vi "RT Main.vi"() -> ()   [LabVIEW 2016]
panel:
  out "dequeued element":i32
  out "elements in queue":i32[](array[numeric])
  out "# elements in queue":i32
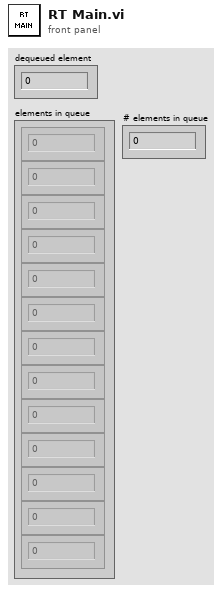
[diagram p1: front panel]
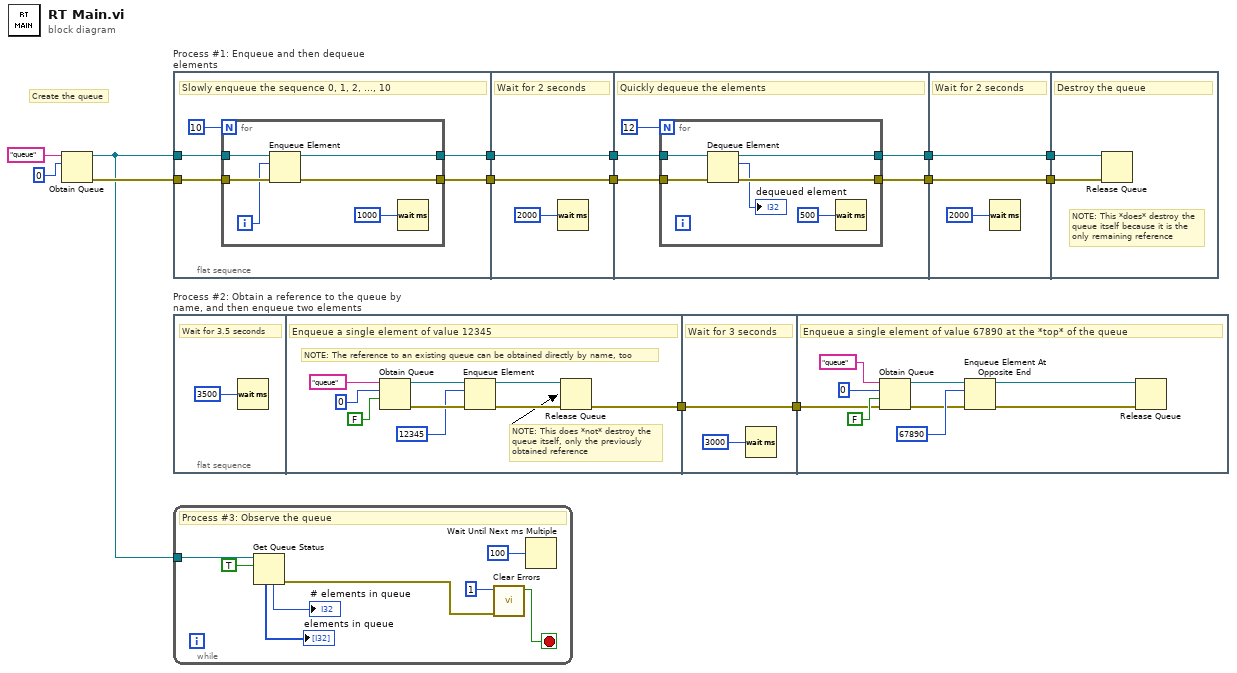
[diagram p0: block diagram]
diagram:
  # "Create the queue"
  n1 = Obtain Queue(name (unnamed)="queue", element data type=0) -> (queue out=w11:refnum<queue>, error out=w12:errorcluster)  [unwired: 3 in, 1 out]
  n2 = flat-sequence "Process #1: Enqueue and then dequeue elements" {
    tunnel: w12 -> [w19]
    tunnel: w11 -> [w17]
    tunnel: [w16] -> w8
    tunnel: [w15] -> w7
    tunnel: w8 -> [w27]
    tunnel: [w27] -> w6
    tunnel: w7 -> [w26]
    tunnel: [w26] -> w5
    tunnel: w6 -> [w29]
    tunnel: w5 -> [w30]
    tunnel: [w32] -> w4
    tunnel: [w31] -> w3
    tunnel: w4 -> [w42]
    tunnel: w3 -> [w41]
    tunnel: [w42] -> w2
    tunnel: [w41] -> w1
    tunnel: w2 -> [w44]
    tunnel: w1 -> [w43]
    frame #0 {
      # "Slowly enqueue the sequence 0, 1, 2, ..., 10"
      n3 = for {
        N: 10 -> [_]
        tunnel: w19 -> [w25]
        tunnel: w17 -> [w24]
        tunnel: [w21] -> w15
        tunnel: [w20] -> w16
        i -> [w23]
        n4 = Enqueue Element(queue=w24, element=w23, error in (no error)=w25) -> (queue out=w20:refnum<queue>, error out=w21:errorcluster)  [unwired: 1 in, 1 out]
        n5 = Wait (ms)(milliseconds to wait=u32 1000 ("millisecond multiple")) -> ()  [unwired: 1 out]
      }
    }
    frame #1 {
      # "Wait for 2 seconds"
      n6 = Wait (ms)(milliseconds to wait=u32 2000 ("millisecond multiple")) -> ()  [unwired: 1 out]
    }
    frame #2 {
      # "Quickly dequeue the elements"
      n7 = for {
        N: 12 -> [_]
        tunnel: [w38] -> w31
        tunnel: [w37] -> w32
        tunnel: w30 -> [w35]
        tunnel: w29 -> [w34]
        n8 = Dequeue Element(queue=w34, error in (no error)=w35) -> (queue out=w37:refnum<queue>, element=→"dequeued element":i32, error out=w38:errorcluster)  [unwired: 1 in, 1 out]
        n9 = Wait (ms)(milliseconds to wait=u32 500 ("millisecond multiple")) -> ()  [unwired: 1 out]
      }
    }
    frame #3 {
      # "Wait for 2 seconds"
      n10 = Wait (ms)(milliseconds to wait=u32 2000 ("millisecond multiple")) -> ()  [unwired: 1 out]
    }
    frame #4 {
      # "NOTE: This *does* destroy the\nqueue itself because it is the\nonly remaining reference"
      # "Destroy the queue"
      n11 = Release Queue(queue=w44, error in (no error)=w43) -> ()  [unwired: 1 in, 3 out]
    }
  }
  n12 = flat-sequence "Process #2: Obtain a reference to the queue by name, and then enqueue two elements" {
    tunnel: [w46] -> w10
    tunnel: w10 -> [w56]
    tunnel: [w56] -> w9
    tunnel: w9 -> [w57]
    frame #0 {
      # "Wait for 3.5 seconds"
      n13 = Wait (ms)(milliseconds to wait=u32 3500 ("millisecond multiple")) -> ()  [unwired: 1 out]
    }
    frame #1 {
      # "NOTE: The reference to an existing queue can be obtained directly by name, too"
      # "NOTE: This does *not* destroy the\nqueue itself, only the previously\nobtained reference"
      # "Enqueue a single element of value 12345"
      n14 = Obtain Queue(name (unnamed)="queue", element data type=0, create if not found? (T)=FALSE) -> (queue out=w50:refnum<queue>, error out=w51:errorcluster)  [unwired: 2 in, 1 out]
      n15 = Enqueue Element(queue=w50, element=12345, error in (no error)=w51) -> (queue out=w47:refnum<queue>, error out=w48:errorcluster)  [unwired: 1 in, 1 out]
      n16 = Release Queue(queue=w47, error in (no error)=w48) -> (error out=w46:errorcluster)  [unwired: 1 in, 2 out]
    }
    frame #2 {
      # "Wait for 3 seconds"
      n17 = Wait (ms)(milliseconds to wait=u32 3000 ("millisecond multiple")) -> ()  [unwired: 1 out]
    }
    frame #3 {
      # "Enqueue a single element of value 67890 at the *top* of the queue"
      n18 = Obtain Queue(name (unnamed)="queue", element data type=0, create if not found? (T)=FALSE, error in (no error)=w57) -> (queue out=w62:refnum<queue>, error out=w61:errorcluster)  [unwired: 1 in, 1 out]
      n19 = Enqueue Element At Opposite End(queue=w62, element=67890, error in (no error)=w61) -> (queue out=w65:refnum<queue>, error out=w64:errorcluster)  [unwired: 1 in, 1 out]
      n20 = Release Queue(queue=w65, error in (no error)=w64) -> ()  [unwired: 1 in, 3 out]
    }
  }
  n21 = while {
    tunnel: w11 -> [w73]
    stop <- w66 stop-if-true
    # "Process #3: Observe the queue"
    n22 = Get Queue Status(queue=w73, return elements? (F)=TRUE) -> (error out=w68:errorcluster, # elements in queue=→"# elements in queue":i32, elements=→"elements in queue":i32[])  [unwired: 1 in, 5 out]
    n23 = call <vilib>:"Clear Errors.vi"("error in (no error)"=w68, "specific error code to clear (0: all)"=1) -> ("specific error cleared?"=w66:bool)  [unwired: 4 in, 1 out]
    n24 = Wait Until Next ms Multiple(millisecond multiple=u32 100) -> ()  [unwired: 1 out]
  }
